vi "DAQ_Input_Slow.vi"() -> ()   [LabVIEW 2014]
uses:
  <vilib>/Platform/TimedLoop/XDataNode/timing_clust.ctl
  <vilib>/Platform/TimedLoop/XDataNode/nitl_modes.ctl
  <vilib>/Platform/TimedLoop/XDataNode/wakeup.ctl
  <vilib>/Analysis/baseanly.llb/Mean (DBL).vi
  <vilib>/FPGAPlugInAG/myRIO-1900/niLvFpga_Open_myRIO-1900.vi
  <vilib>/rvi/interface/common/dynamic/niFpgaDynamicAddResources.vi
  <vilib>/Utility/error.llb/Error Cluster From Error Code.vi
  <vilib>/rvi/errors/niLvFpgaAdjustHostInterfaceError.vi
  <vilib>/FPGAPlugInAG/Dynamic/niLvFpga_Close_Dynamic.vi
  <vilib>/rvi/interface/nirviOpenFPGA/nirviOpenFPGA.xnode
  FPGA Bitfiles/FirstTrial_FPGATarget_FPGAMainInputMeasurement_10V.lvbitx
  <vilib>/rvi/interface/nirviReadWriteControl/nirviReadWriteControl.xnode
  <vilib>/rvi/interface/nirviMethod/nirviMethod.xnode
  <vilib>/Platform/TimedLoop/XDataNode/XDataNode.xnode
  <vilib>/rvi/interface/nirviCloseFPGA/nirviCloseFPGA.xnode
  <vilib>/rvi/errors/niLvFpgaMergeErrorWithErrorCode.vi
  <vilib>/rvi/interface/Simulation/niFpgaSimulationCallBeginRW.vi
  <vilib>/Platform/TimedLoop/XDataNode/XDNodeRunTimeDep.lvlib
  <vilib>/Analysis/NI_AALBase.lvlib
  <vilib>/FPGAPlugInAG/Dynamic/niLvFpga_ReadFifo_Dynamic.vi
  NiFpgaLv.dll
  <vilib>/FPGAPlugInAG/Dynamic/niLvFpga_StartFifo_Dynamic.vi
  <vilib>/FPGAPlugInAG/Dynamic/niLvFpga_StopFifo_Dynamic.vi
panel:
  in  "System ID?":bool
  in  "Acquisitions":T1(tab)=enum."Recorded"
  out "Real Time Actuation Mean Chart":dbl(graph)=2.577495574951172
  out "Real Time Measurement Mean Chart":dbl(graph)=2.4726343154907227
  out "Measurement Data":i16[](array[numeric])=[754, 1268, 1779, 2292, 2798, 3300, 3794, 4083, 4089, 4094, 4094, 4095, 4093, 4095, 4094, 4095, 4094, 4095, 4093, 4095, 4093, 4094, 4093, 4095, 4093, 4095, 4093, 4095, 4093, 4095, 4093, 4095, 4093, 4095, 4093, 4095, 4092, 4095, 4092, 4095, 4092, 4095, 4092, 4095, 4093, 4095, 4094, 4095, 4094, 4095, 4094, 4095, 4094, 4095, 4095, 4095, 4094, 4095, 4094, 4094, 3947, 3428, 2884, 2343, 1812, 1284, 760, 250, 10, 8, 5, 5, 4, 4, 5, 5, 5, 5, 5, 4, 5, 5, 5, 4, 5, 4, 5, 5, 5, 5, 5, 5, 5, 4, 5, 5, 5, 5, 4, 5, 4, 5, 5, 5, 5, 4, 4, 5, 5, 5, 5, 5, 4, 5, 5, 5, 4, 5, 5, 5, 5, 5, 5, 136, 636, 1150, 1662, 2175, 2682, 3186, 3680, 4088, 4089, 4093, 4093, 4095, 4094, 4095, 4093, 4095, 4094, 4095, 4093, 4094, 4093, 4095, 4093, 4094, 4093, 4095, 4093, 4095, 4094, 4095, 4094, 4095, 4093, 4095, 4093, 4095, 4093, 4095, 4092, 4095, 4092, 4095, 4092, 4095, 4093, 4095, 4094, 4095, 4093, 4095, 4094, 4095, 4094, 4095, 4094, 4095, 4094, 4095, 4094, 4095, 4060, 3570, 3029, 2485, 1952, 1423, 897, 382, 4, 9, 6, 5, 4, 4, 5, 5, 5, 5, 4, 4, 4, 5, 5, 4, 5, 5, 5, 5, 5, 5, 5, 5, 4, 5, 5, 5, 5, 5, 5, 4, 5, 5, 5, 4, 4, 4, 5, 5, 5, 5, 5, 5, 5, 5, 5, 5, 5, 4, 5, 5, 5, 5, 5, 7, 500, 1013, 1526, 2037, 2548, 3052, 3550, 4034]
  out "Actuation Data":i16[](array[numeric])=[4095, 4095, 4095, 4095, 4095, 4095, 4095, 4095, 4095, 4095, 4095, 4095, 4095, 4095, 4095, 4095, 4095, 4095, 4095, 4095, 4095, 4095, 4095, 4095, 4095, 4095, 4095, 4095, 4095, 4095, 4095, 4095, 4095, 4095, 4095, 4095, 4095, 4095, 4095, 4095, 4095, 4095, 4095, 4095, 4095, 4095, 4095, 4095, 4095, 4095, 4095, 4095, 4095, 4095, 4095, 4095, 4095, 4095, 4095, 0, 0, 0, 0, 0, 0, 0, 0, 0, 0, 0, 0, 0, 0, 0, 0, 0, 0, 0, 0, 0, 0, 0, 0, 0, 0, 0, 0, 0, 0, 0, 0, 0, 0, 0, 0, 0, 0, 0, 0, 0, 0, 0, 0, 0, 0, 0, 0, 0, 0, 0, 0, 0, 0, 0, 0, 0, 0, 0, 0, 0, 0, 4095, 4095, 4095, 4095, 4095, 4095, 4095, 4095, 4095, 4095, 4095, 4095, 4095, 4095, 4095, 4095, 4095, 4095, 4095, 4095, 4095, 4095, 4095, 4095, 4095, 4095, 4095, 4095, 4095, 4095, 4095, 4095, 4095, 4095, 4095, 4095, 4095, 4095, 4095, 4095, 4095, 4095, 4095, 4095, 4095, 4095, 4095, 4095, 4095, 4095, 4095, 4095, 4095, 4095, 4095, 4095, 4095, 4095, 4095, 4095, 4095, 4095, 0, 0, 0, 0, 0, 0, 0, 0, 0, 0, 0, 0, 0, 0, 0, 0, 0, 0, 0, 0, 0, 0, 0, 0, 0, 0, 0, 0, 0, 0, 0, 0, 0, 0, 0, 0, 0, 0, 0, 0, 0, 0, 0, 0, 0, 0, 0, 0, 0, 0, 0, 0, 0, 0, 0, 0, 0, 0, 0, 0, 0, 0, 4095, 4095, 4095, 4095, 4095, 4095, 4095, 4095, 4095, 4095, 4095]
  out "Mean Measurement":dbl=2.4726343154907227 format="%0.2f"
  out "Mean Acatuation":dbl=2.577495574951172 format="%0.2f"
  out "Elements Remaining":u32=192
  out "Actuation Graph":waveform(i16)(graph)={"t0"=timestamp(0 s since 1904-01-01), "dt"=2.0, "Y"=array[3392 elements]}
  out "Measurement Graph":waveform(i16)(graph)={"t0"=timestamp(0 s since 1904-01-01), "dt"=2.0, "Y"=array[3520 elements]}
  out "Data File Path":path=path "c:/ni-rt/startup/03_11_16_04:11 PMTrial.csv"
  out "Sample Each Cycle":i32[](array[numeric])=[0, 0, 512, 960, 576, 384, 256, 192, 256, 256]
  out "Total Data Points":i32=3392
  out "Actuation Graph 2":waveform(dbl)(graph)
  in  "Settings":T2(tab)
  in  "Actuation Period (muS)":u32=8
  in  "Acquisition Period (muS)":u32=8
  in  "RT Period(muS)":i64=500
  in  "Recording Time (muS)":i64=5000
  in  "Signal Control":T3={"Mode"=enum."Square Wave", "Frequency (Periods/tick)"=0.0001005989033728838, "Phase (period)"=0.0} {"Frequency (Periods/tick)" format="%#_6f"}
  out "Frequency (kHz)":dbl=4.023956134915352
  in  "High Pass?":bool
  in  "Low Pass?":bool
  in  "Data File Name Label":string="Trial"
  in  "Current Source Resistance (ohm)":dbl=20.0
  in  "INA Resistance (ohm)":dbl=20.0
  in  "Continuous?":bool
  in  "Log Data?":bool
  out "Logging Progress":dbl(slide) scale=0.0..100.0
  out "Logging?":bool
  out "Finished Late? [i-1]":bool
  in  "stop":bool
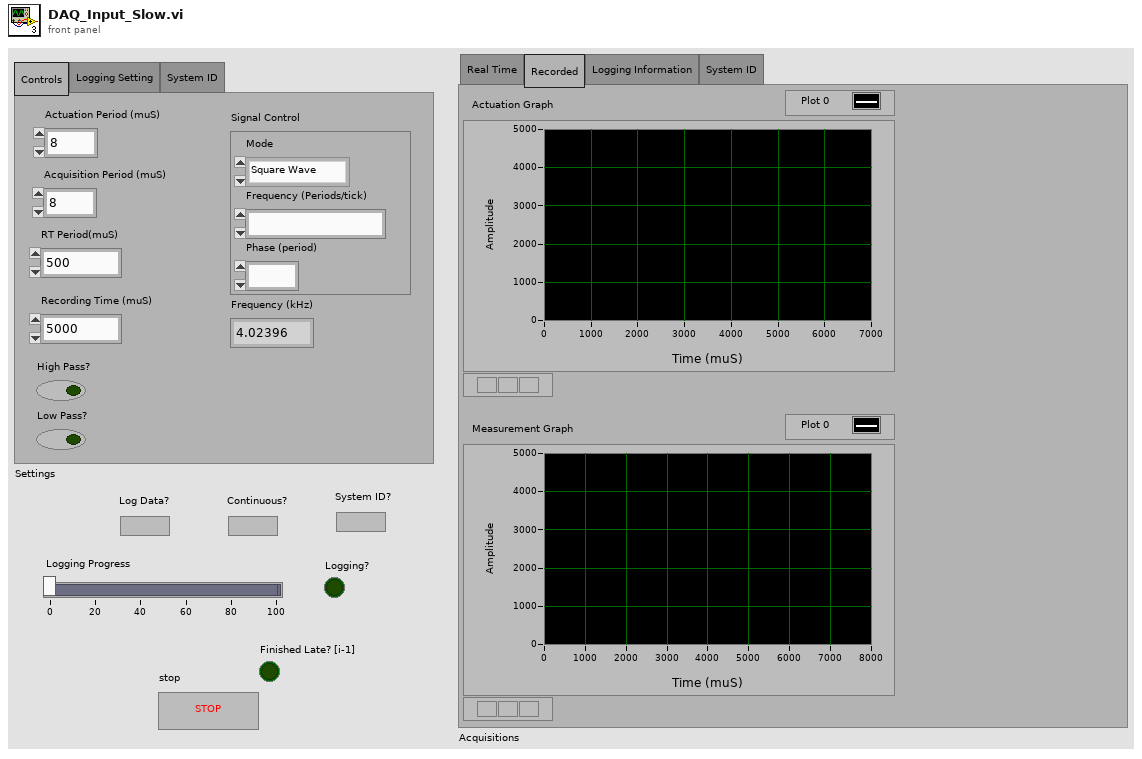
[diagram p1: front panel]
types:
  T1 = enum32{"Real Time", "Recorded", "Logging Information", "System ID"}
  T2 = enum32{"Controls", "Logging Setting", "System ID"}
  T3 = cluster{"Mode":enum16{"Square Wave", "Sine Wave", "White Noise", "Stochastic"}, "Frequency (Periods/tick)":fxp<+,32,0>, "Phase (period)":fxp<+,32,0>}
  T4 = typedef "XDNodeRunTimeDep.lvlib/timing_clust.ctl" = cluster{"Expected End [f-1]":u64, "Actual End [f-1]":u64, "Finished Late? [f-1]":bool, "Expected End [i-1]":u64, "Actual End [i-1]":u64, "Finished Late? [i-1]":bool, "Expected Start [i]":u64, "Actual Start [i]":u64, "Expected Start [f]":u64, "Actual Start [f]":u64, "Source Name":string, "Structure Name":string, "Period":i64, "Deadline":i64, "Offset":i64, "Start":i64, "Priority":i32, "Timeout":i32, "Mode":T5, "Wakeup Reason":T6, "Error":errorcluster, "Source Type":string, "Secondary Source Type":string, "Global End Time":u64, "Global Start Time":u64, "Frame Duration":u64, "Iteration Duration":u64, "Assigned CPU":i32, "I/O Scan Engine Mode":u32}
  T5 = typedef "XDNodeRunTimeDep.lvlib/nitl_modes.ctl" = enum32{"No Change", "Process missed periods, maintain original phase", "Discard missed periods, maintain original phase", "Process missed periods, ignore original phase", "Discard missed periods, ignore original phase"}
  T6 = typedef "XDNodeRunTimeDep.lvlib/wakeup.ctl" = enum32{"Normal", "Aborted", "Asynchronous wakeup", "Timing source error", "Timed loop error", "Timeout"}
  T7 = enum16{"open", "replace", "create", "open or create", "replace or create", "replace or create with confirmation"}
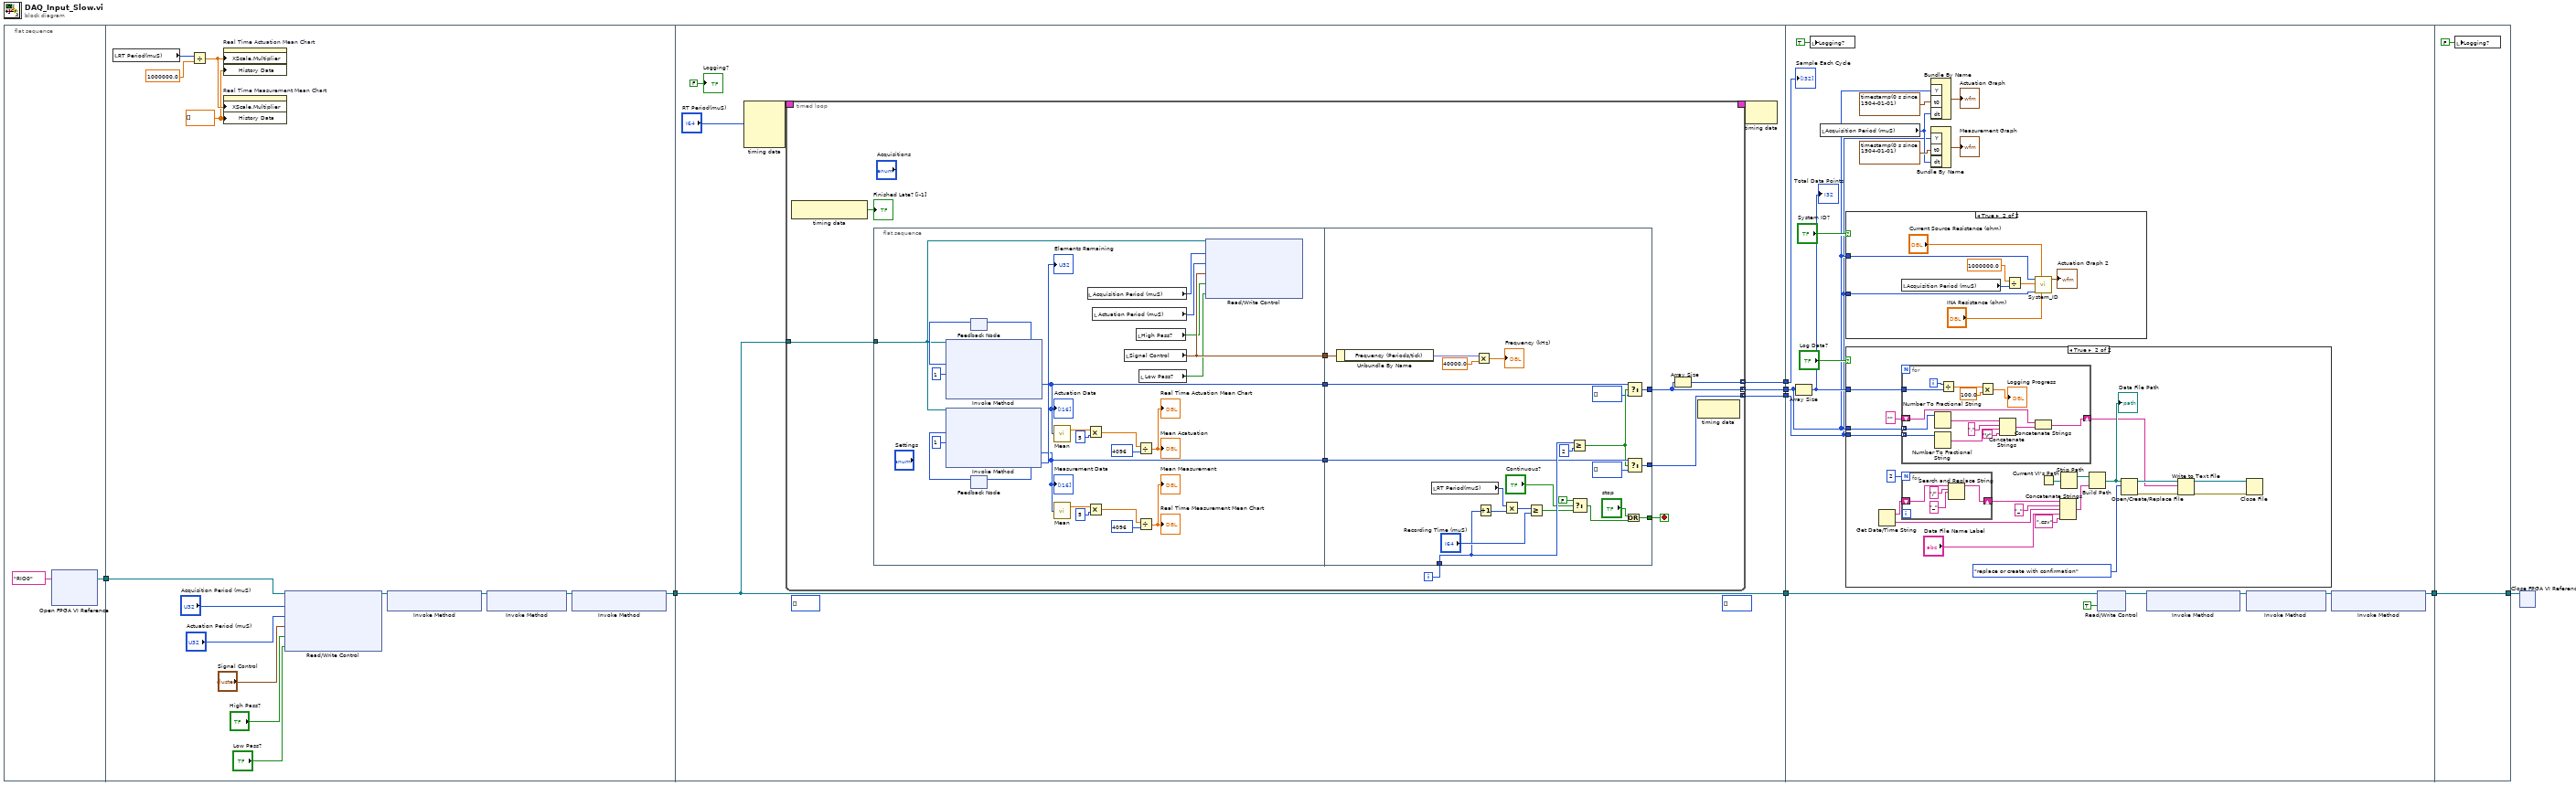
[diagram p0: block diagram]
diagram:
  n1 = flat-sequence {
    tunnel: [w9] -> w6
    tunnel: w6 -> [w17]
    tunnel: [w12] -> w5
    tunnel: w5 -> [w29]
    tunnel: [w29] -> w8
    tunnel: [w28] -> w4
    tunnel: [w27] -> w3
    tunnel: [w25] -> w1
    tunnel: w8 -> [w113]
    tunnel: w4 -> [w98]
    tunnel: w3 -> [w97]
    tunnel: [w100] -> w2
    tunnel: w1 -> [w109]
    tunnel: [w163] -> w7
    tunnel: w2 -> [w163]
    frame #0 {
      n2 = xnode "Open FPGA VI Reference"("resource name"=tag "RIO0") -> ("FPGA VI Reference Out"=w9:refnum<k20>)  [unwired: 1 in, 1 out]
    }
    frame #1 {
      w15 = dbl[] [] ("History Data")
      n3 = local read "RT Period(muS)"() -> (w20:i64)
      n4 = Divide(x=w20, y=1000000.0 ("x")) -> (x/y=w16:dbl)
      n5 = property on="Real Time Actuation Mean Chart" class="WFChart (strict)"("XScale.Multiplier"=w16, "History Data"=w15) -> ()  [unwired: 2 in, 2 out]
      n6 = property on="Real Time Measurement Mean Chart" class="WFChart (strict)"("XScale.Multiplier"=w16, "History Data"=w15) -> ()  [unwired: 2 in, 2 out]
      n7 = xnode "Read/Write Control"("FPGA VI Reference In"=w17, "Acquisition Period (muS)"="Acquisition Period (muS)", "Actuation Period (muS)"="Actuation Period (muS)", "Cluster"="Signal Control", "High Pass?"="High Pass?", "Low Pass?"="Low Pass?") -> ("FPGA VI Reference Out"=w19:refnum<k20>)  [unwired: 1 in, 1 out]
      n8 = xnode "Invoke Method"("FPGA VI Reference In"=w19) -> ("FPGA VI Reference Out"=w18:refnum<k20>)  [unwired: 1 in, 1 out]
      n9 = xnode "Invoke Method"("FPGA VI Reference In"=w18) -> ("FPGA VI Reference Out"=w11:refnum<k20>)  [unwired: 1 in, 1 out]
      n10 = xnode "Invoke Method"("FPGA VI Reference In"=w11) -> ("FPGA VI Reference Out"=w12:refnum<k20>)  [unwired: 1 in, 1 out]
    }
    frame #2 {
      (unwired) i16[] []
      (unwired) i16[] []
      n11 = node-c288("RT Period(muS)") -> (w32:T4)  [unwired: 3 in]
      n12 = timed-loop {
        tunnel: w29 -> [w41]
        timing: w32 -> [_]
        timing-out: [_] -> w31
        tunnel: [w35] -> w28 mode=concatenating
        tunnel: [w40] -> w27 mode=concatenating
        tunnel: [w34] -> w25 mode=indexing
        i -> [w37]
        stop <- w36 stop-if-true
        n13 = node-c288() -> (→"Finished Late? [i-1]":bool)  [unwired: 1 in]
        n14 = flat-sequence {
          tunnel: w41 -> [w52]
          tunnel: [w49] -> w39
          tunnel: [w48] -> w38
          tunnel: [w45] -> w33
          tunnel: [w83] -> w40
          tunnel: [w76] -> w35
          tunnel: w39 -> [w77]
          tunnel: w38 -> [w80]
          tunnel: w37 -> [w82]
          tunnel: [w84] -> w36
          tunnel: w33 -> [w74]
          frame #0 {
            n15 = feedback #1() -> (w58:u32)  [unwired: 1 in]
            n16 = xnode "Invoke Method"("FPGA VI Reference In"=w52, "Number of Elements"=w58, "Timeout (ms)"=1) -> ("Data"=w49:i16[], "Elements Remaining"=w57:u32)  [unwired: 1 in, 2 out]
            "Actuation Data" <- w49
            n17 = feedback-in #1(w57) -> ()
            n18 = feedback #2() -> (w65:u32)  [unwired: 1 in]
            n19 = xnode "Invoke Method"("FPGA VI Reference In"=w52, "Number of Elements"=w65, "Timeout (ms)"=1) -> ("Data"=w48:i16[], "Elements Remaining"=w66:u32)  [unwired: 1 in, 2 out]
            "Measurement Data" <- w48
            "Elements Remaining" <- w66
            n20 = feedback-in #2(w66) -> ()
            n21 = call-poly <vilib>:"Mean.vi"("X"=w49) -> ("mean"=w53:dbl)  [unwired: 1 out]
            n22 = call-poly <vilib>:"Mean.vi"("X"=w48) -> ("mean"=w60:dbl)  [unwired: 1 out]
            n23 = local read "Acquisition Period (muS)"() -> (w51:u32)
            n24 = Multiply(x=w53, y=u16 5) -> (x*y=w54:dbl)
            n25 = Multiply(x=w60, y=u16 5) -> (x*y=w61:dbl)
            n26 = local read "Actuation Period (muS)"() -> (w50:u32)
            n27 = local read "Signal Control"() -> (w45:T3)
            n28 = local read "High Pass?"() -> (w44:bool)
            n29 = Divide(x=w54, y=u16 4096) -> (x/y=→"Real Time Actuation Mean Chart" →"Mean Acatuation":dbl)
            n30 = Divide(x=w61, y=u16 4096) -> (x/y=→"Mean Measurement" →"Real Time Measurement Mean Chart":dbl)
            n31 = local read "Low Pass?"() -> (w43:bool)
            n32 = xnode "Read/Write Control"("FPGA VI Reference In"=w52, "Acquisition Period (muS)"=w51, "Actuation Period (muS)"=w50, "Cluster"=w45, "High Pass?"=w44, "Low Pass?"=w43) -> ()  [unwired: 1 in, 2 out]
          }
          frame #1 {
            n33 = Unbundle By Name(w74) -> ("Frequency (Periods/tick)"=w72:fxp<+,32,0>)
            n34 = local read "RT Period(muS)"() -> (w86:i64)
            n35 = Multiply(x=w72, y=40000.0) -> (x*y=→"Frequency (kHz)":dbl)
            n36 = Increment(x=w82) -> (x+1=w88:i32)
            n37 = Multiply(x=w86, y=w88) -> (x*y=w87:i64)
            n38 = Greater Or Equal?(x=w87, y="Recording Time (muS)") -> (x >= y?=w69:bool)
            n39 = Greater Or Equal?(x=w82, y=2) -> (x >= y?=w78:bool)
            n40 = Select(t=FALSE, s="Continuous?", f=w69) -> (s? t:f=w68:bool)
            n41 = Or(x="stop", y=w68) -> (x .or. y?=w84:bool)
            n42 = Select(t=w77, s=w78, f=i16[] []) -> (s? t:f=w76:i16[])
            n43 = Select(t=w80, s=w78, f=i16[] []) -> (s? t:f=w83:i16[])
          }
        }
        n44 = Array Size(array=w35) -> (size(s)=w34:i32)
        n45 = node-c288() -> ()  [unwired: 1 in, 1 out]
      }
      n46 = node-c288(w31) -> ()  [unwired: 1 out]
      "Logging?" <- FALSE ("Logging?")
    }
    frame #3 {
      n47 = Array Size(array=w98) -> (size(s)=w108:i32)
      "Total Data Points" <- w108
      n48 = local write "Logging?"(TRUE ("Logging?")) -> ()
      n49 = local read "Acquisition Period (muS)"() -> (w102:u32)
      n50 = case shown="True" "System ID?" {
        tunnel: w98 -> [_ w122]
        tunnel: w97 -> [_ w121]
        frame False {
        }
        frame True {
          n51 = local read "Acquisition Period (muS)"() -> (w117:u32)
          n52 = Divide(x=1000000.0, y=w117) -> (x/y=w115:dbl)
          n53 = call "System_ID.vi"("INA Resistance (ohm)"="INA Resistance (ohm)", "Current Source Resistance (ohm)"="Current Source Resistance (ohm)", "Input Y"=w121, "Sample_Frequency (Hz)"=w115, "Input X"=w122) -> ("Actuation Graph"=→"Actuation Graph 2":waveform(dbl))  [unwired: 3 in, 3 out]
        }
      }
      n54 = case shown="True" "Log Data?" {
        tunnel: w97 -> [_ w128]
        tunnel: w98 -> [_ w127]
        tunnel: w108 -> [_ w126]
        frame False {
        }
        frame True {
          n55 = Get Date/Time String() -> (date string=w136:string, time string=w132:string)  [unwired: 3 in]
          n56 = for {
            shift-right: [w154] -> w125
            shift-left: "" -> [w153]
            tunnel: w128 -> [w150] mode=indexing
            tunnel: w127 -> [w149] mode=indexing
            tunnel: w126 -> [w145]
            i -> [w144]
            n57 = Number To Fractional String(number=w149) -> (F-format string=w152:string)  [unwired: 3 in]
            n58 = Number To Fractional String(number=w150) -> (F-format string=w156:string)  [unwired: 3 in]
            n59 = Divide(x=w144, y=w145) -> (x/y=w148:dbl)
            n60 = Multiply(x=w148, y=100.0) -> (x*y=→"Logging Progress":dbl)
            n61 = Concatenate Strings(w152, "," ("string"), w156, "\r") -> (w155:string)
            n62 = Concatenate Strings(w153, w155) -> (w154:string)
          }
          n63 = for {
            N: 2 -> [_]
            shift-right: [w159] -> w134
            shift-left: w136 -> [w158]
            n64 = Search and Replace String(input string=w158, search string="/", replace string="_" ("replace string (\"\")")) -> (result string=w159:string)  [unwired: 5 in, 3 out]
          }
          n65 = Current VI's Path() -> (path=w138:path)
          n66 = Concatenate Strings(w134, "_" ("replace string (\"\")"), w132, "Data File Name Label", ".csv" ("replace string (\"\")")) -> (w131:string)
          n67 = Strip Path(path=w138) -> (stripped path=w137:path)  [unwired: 1 out]
          n68 = Build Path(base path=w137, name or relative path=w131) -> (appended path=w130:path)
          "Data File Path" <- w130
          n69 = Open/Create/Replace File(file path (use dialog)=w130, operation (0:open)=T7."replace or create with confirmation") -> (refnum out=w142:refnum<file>, error out=w141:errorcluster)  [unwired: 4 in, 1 out]
          n70 = Write to Text File(file (use dialog)=w142, text=w125, error in=w141) -> (refnum out=w140:refnum<file>, error out=w139:errorcluster)  [unwired: 1 in, 1 out]
          n71 = Close File(refnum=w140, error in=w139) -> ()  [unwired: 2 out]
        }
      }
      n72 = Bundle By Name("Y"=w98, "t0"=timestamp(0 s since 1904-01-01), "dt"=w102) -> (→"Actuation Graph":waveform(i16))  [unwired: 1 in]
      n73 = Bundle By Name("Y"=w97, "t0"=timestamp(0 s since 1904-01-01), "dt"=w102) -> (→"Measurement Graph":waveform(i16))  [unwired: 1 in]
      n74 = xnode "Read/Write Control"("FPGA VI Reference In"=w113, "stop"=TRUE) -> ("FPGA VI Reference Out"=w112:refnum<k20>)  [unwired: 1 in, 1 out]
      n75 = xnode "Invoke Method"("FPGA VI Reference In"=w112) -> ("FPGA VI Reference Out"=w114:refnum<k20>)  [unwired: 1 in, 1 out]
      n76 = xnode "Invoke Method"("FPGA VI Reference In"=w114) -> ("FPGA VI Reference Out"=w101:refnum<k20>)  [unwired: 1 in, 1 out]
      n77 = xnode "Invoke Method"("FPGA VI Reference In"=w101) -> ("FPGA VI Reference Out"=w100:refnum<k20>)  [unwired: 1 in, 1 out]
      "Sample Each Cycle" <- w109
    }
    frame #4 {
      n78 = local write "Logging?"(FALSE ("Logging?")) -> ()
    }
  }
  n79 = xnode "Close FPGA VI Reference"("FPGA VI Reference In"=w7) -> ()  [unwired: 1 in, 1 out]
